vi "IMU Sensor Data.vi"() -> ()   [LabVIEW 2015]
panel:
  out "IMU Yaw":dbl
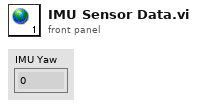
[diagram p1: front panel]
diagram:
